vi "Get Query HTML.vi"(9 "Module Settings":T1(array[cluster]), 10 "Assembly Tray Region":i32, 11 "Tray":i32) -> (3 "Module Array":refnum<class "Module.lvclass">[](array[class]))   [LabVIEW 2019, in "Module.lvclass"]
uses:
  Module.lvclass
  Module.lvclass/Module.ctl
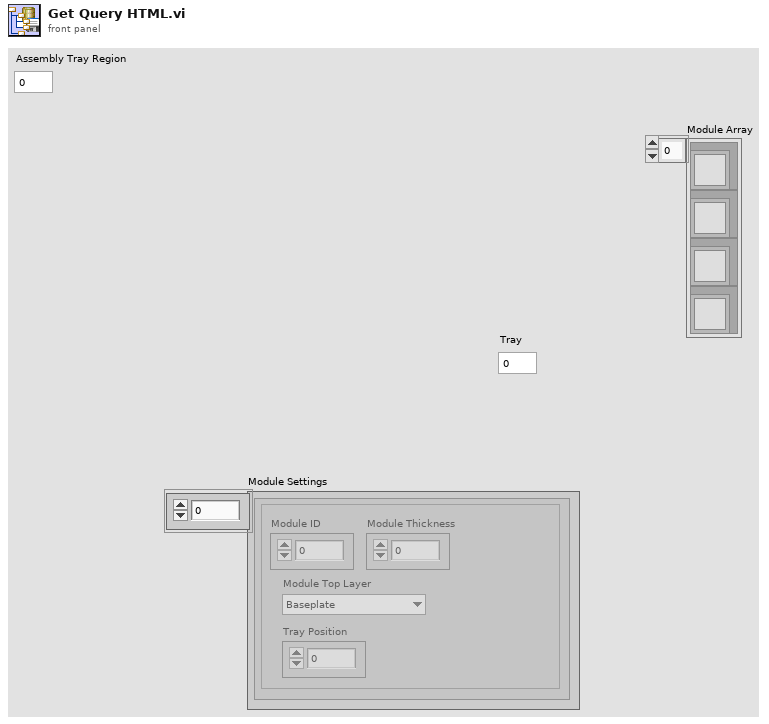
[diagram p1: front panel]
types:
  T1 = cluster{"Module ID":dbl, "Module Thickness":dbl, "Module Top Layer":enum16{"Baseplate", "Kapton", "Sensor", "PCB"}, "Tray Position":dbl}[]
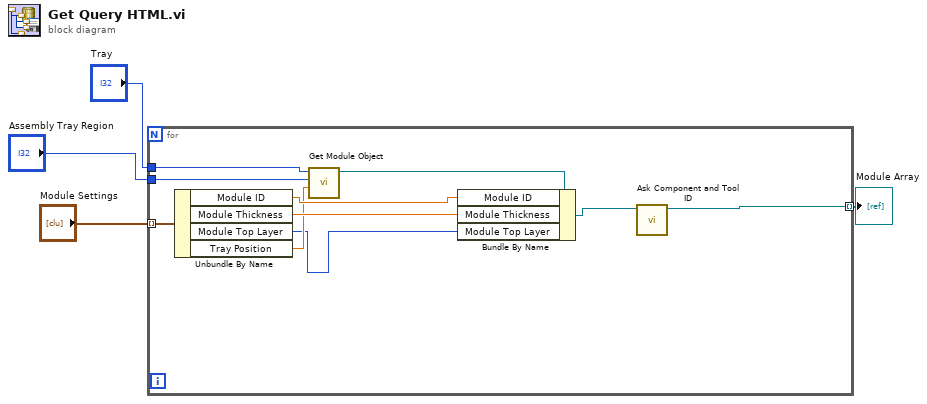
[diagram p0: block diagram]
diagram:
  n1 = for {
    tunnel: "Tray" -> [w14]
    tunnel: [w13] -> w4 mode=indexing
    tunnel: "Module Settings" -> [w11] mode=indexing
    tunnel: "Assembly Tray Region" -> [w8]
    n2 = Unbundle By Name(w11) -> ("Module ID"=w10:dbl, "Module Thickness"=w9:dbl, "Module Top Layer"=w5:enum16{"Baseplate", "Kapton", "Sensor", "PCB"}, "Tray Position"=w7:dbl)
    n3 = call "Get Module Object.vi"("Assembly Tray Position"=w7, "Assembly Tray Region"=w8, "Assembly Tray Number"=w14) -> ("Module.lvclass"=w6:refnum<class "Module.lvclass">)  [unwired: 7 in, 1 out]
    n4 = Bundle By Name(cluster=w6, "Module ID"=w10, "Module Thickness"=w9, "Module Top Layer"=w5) -> (w12:refnum<class "Module.lvclass">)
    n5 = call "Ask Component and Tool ID.vi"("Module In"=w12) -> ("Module Out"=w13:refnum<class "Module.lvclass">)  [unwired: 10 in]
  }
  "Module Array" <- w4
